vi "Configure Compliance Limit Test.vi"(7 "Enable Compliance Limit Test  (T:Enable)":bool=TRUE, 8 "error in (no error)":errorcluster, 9 "Compliance Test Failure I/O Output (0)":u32, 10 "Compliance Test Failure Condition (0: Out of Compliance)":u16(ring) items=["Out of Compliance", "In Compliance"], 11 "VISA resource name":refnum<visa-resource-name>) -> (0 "error out":errorcluster, 3 "VISA resource name out":refnum<visa-resource-name>)   [LabVIEW 2019, in "Keithley 24XX.lvlib"]
doc: "Configures the compliance and contact check limit tests. These tests correspond to tests number 1 and 4, and cannot be set with the Configure Specific Limit Test VI.\n\n<B>Note:</B> The contact check limit test is optional, and therefore may not be supported on your device."
uses:
  Keithley 24XX.lvlib
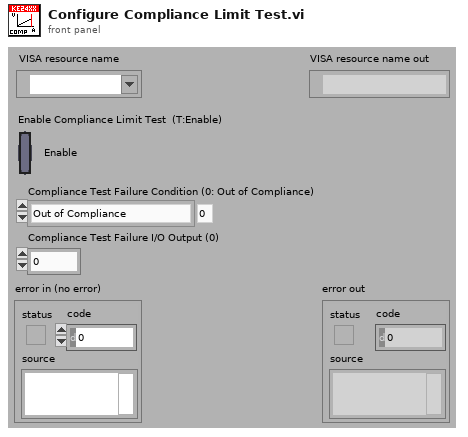
[diagram p1: front panel]
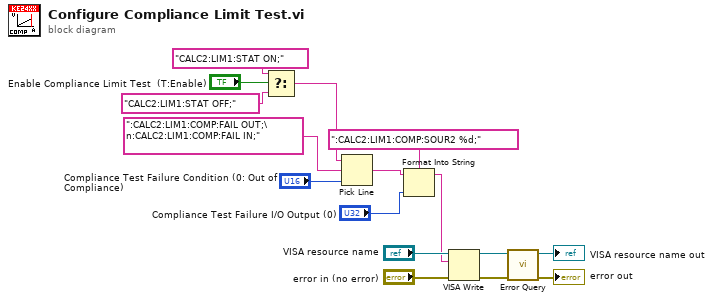
[diagram p0: block diagram]
diagram:
  n1 = Select(t="CALC2:LIM1:STAT ON;", s="Enable Compliance Limit Test  (T:Enable)", f="CALC2:LIM1:STAT OFF;") -> (s? t:f=w12:string)
  n2 = Pick Line(string ("")=w12, multi-line string=":CALC2:LIM1:COMP:FAIL OUT;\n:CALC2:LIM1:COMP:FAIL IN;", line index="Compliance Test Failure Condition (0: Out of Compliance)") -> (output string=w11:string)
  n3 = Format Into String(format string=":CALC2:LIM1:COMP:SOUR2 %d;", initial string=w11, "Compliance Test Failure I/O Output (0)") -> (resulting string=w6:string)  [unwired: 1 in, 1 out]
  n4 = VISA Write(VISA resource name="VISA resource name", write buffer=w6, error in (no error)="error in (no error)") -> (VISA resource name out=w4:refnum<visa-resource-name>, error out=w5:errorcluster)  [unwired: 1 out]
  n5 = call "Error Query.vi"("error in (no error)"=w5, "VISA resource name"=w4) -> ("error out"=→"error out":errorcluster, "VISA resource name out"=→"VISA resource name out":refnum<visa-resource-name>)  [unwired: 6 in, 2 out]
